vi "RequestPulse.vi"(8 "error in (no error)":errorcluster, 11 "ZanClass in":refnum<class "ZanClass.lvclass">) -> (0 "error out":errorcluster, 2 "Pulse":dbl, 3 "ZanClass out":refnum<class "ZanClass.lvclass">)   [LabVIEW 2019, in "ZanClass.lvclass"]
uses:
  ZanClass.lvclass
  LLB/zmotion/zaux/zauxdll.lvlib
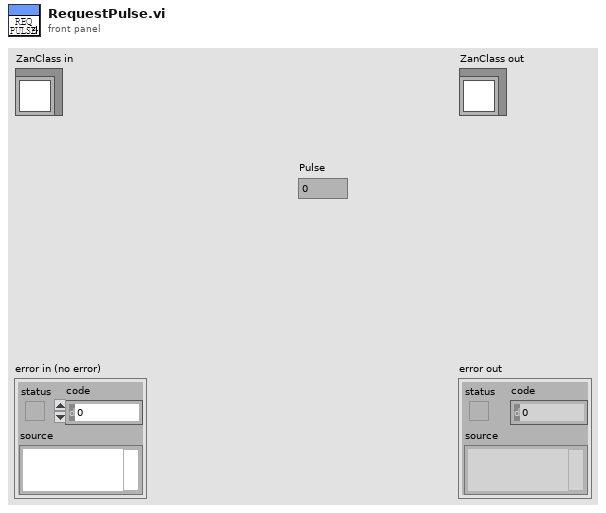
[diagram p1: front panel]
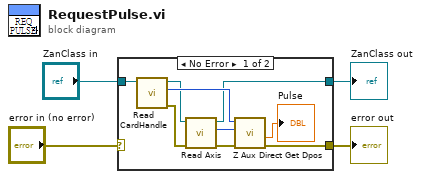
[diagram p0: block diagram]
diagram:
  n1 = case shown="No Error" "error in (no error)" {
    selector: "error in (no error)" -> [_ w14]
    tunnel: "ZanClass in" -> [w13 w15]
    tunnel: [w9 w15] -> w2
    tunnel: [w6 w14] -> w1
    frame No Error {
      n2 = call-dynamic "Read CardHandle.vi"("AxisCard in"=w13) -> ("error out"=w8:errorcluster, "CardHandle"=w12:i32, "AxisCard out"=w11:refnum<class "ZanClass.lvclass">)  [unwired: 8 in]
      n3 = call-dynamic "Read Axis.vi"("error in (no error)"=w8, "AxisCard in"=w11) -> ("error out"=w7:errorcluster, "Axis"=w10:u32, "AxisCard out"=w9:refnum<class "ZanClass.lvclass">)  [unwired: 7 in]
      n4 = call "Z Aux Direct Get Dpos.vi"("error in (no error)"=w7, "iaxis"=w10, "handle"=w12) -> ("error out"=w6:errorcluster, "pfValue out"=→"Pulse":sgl)  [unwired: 5 in, 2 out]
    }
    frame Error {
    }
  }
  "error out" <- w1
  "ZanClass out" <- w2
